vi "Import Configuration and Add Messages.vi"() -> ()   [LabVIEW 2020]
uses:
  <vilib>/addons/VeriStand Custom Device Scripting APIs/Instrument Addon/API/TypeDefs/Message Settings.ctl
  <vilib>/addons/VeriStand Custom Device Scripting APIs/Instrument Addon/API/TypeDefs/Protection Types.ctl
  <vilib>/addons/VeriStand Custom Device Scripting APIs/Instrument Addon/API/TypeDefs/Single Channel Format Settings.ctl
  <vilib>/addons/VeriStand Custom Device Scripting APIs/Instrument Addon/API/TypeDefs/Command Settings.ctl
  <vilib>/NI VeriStand/Custom Device API/Custom Device Item Ref.ctl
  <vilib>/addons/VeriStand Custom Device Scripting APIs/Instrument Addon/API/TypeDefs/Padding.ctl
  <vilib>/addons/VeriStand Custom Device Scripting APIs/Instrument Addon/API/TypeDefs/Array Type Cast Settings.ctl
  <vilib>/addons/VeriStand Custom Device Scripting APIs/Instrument Addon/API/TypeDefs/Array Element.ctl
  <vilib>/addons/VeriStand Custom Device Scripting APIs/Instrument Addon/Shared Directory/Type Cast Type.ctl
  <vilib>/addons/VeriStand Custom Device Scripting APIs/Instrument Addon/Shared Directory/Endian.ctl
  <vilib>/addons/VeriStand Custom Device Scripting APIs/Instrument Addon/API/Channels/Create Global MetaData Channel - Array - Type Cast.vi
  <vilib>/addons/VeriStand Custom Device Scripting APIs/Instrument Addon/API/Messages/Create Message - Value Change & Trigger.vi
  <vilib>/addons/VeriStand Custom Device Scripting APIs/Instrument Addon/API/Channels/Create MetaData Channel - Single Channel - Format.vi
  <vilib>/addons/VeriStand Custom Device Scripting APIs/Instrument Addon/API/Instrument Addon Scripting API.lvlib
  <vilib>/NI VeriStand/Custom Device API/Custom Device API.lvlib
  <vilib>/addons/VeriStand Custom Device Scripting APIs/Instrument Addon/Shared Directory/Instrument Addon Shared.lvlib
panel:
  in  "Configuration File to Import":path=path "Exported Configuration.dat"
  in  "Output System Definition File":path=path "System Definition Files/Import and Add Messages.nivssdf"
  in  "Input System Definition File":path=path "System Definition Files/Base.nivssdf"
  # "Overview: Demonstrate how to create an Instrument Addon Custom Device from a previously exported configuration and add additional messages and channels.\n\nNote: Must first run Basic Example.vi to generate the exported configuration .dat file used by this example.\n\nThe VI executes the following steps:\n1. Loads the exported configuration file from Basic Example.vi to create an Instrument Addon Custom Device with the same configuration.\n2. Adds a Global MetaData Channel and another message.\n3. For the new message, adds a Command Section and a MetaData Channel.\n4. Creates two linked channels by assigning the MetaData Channel refnum and the Global MetaData Channel refnum to two variable names in the command.\n5. Save System Definition file at the specification location.\n\nInstructions:\n1. Browse to the system definition file to be used as input.\n2. Browse to a path to save the system definition file as output. This may be the same as the input file.\n3. Browse to a path to import the previously exported custom device configuration from Basic Example.vi\n4. Run the VI and verify its results."
  # "System Definition Files"
  # "Configuration Files"
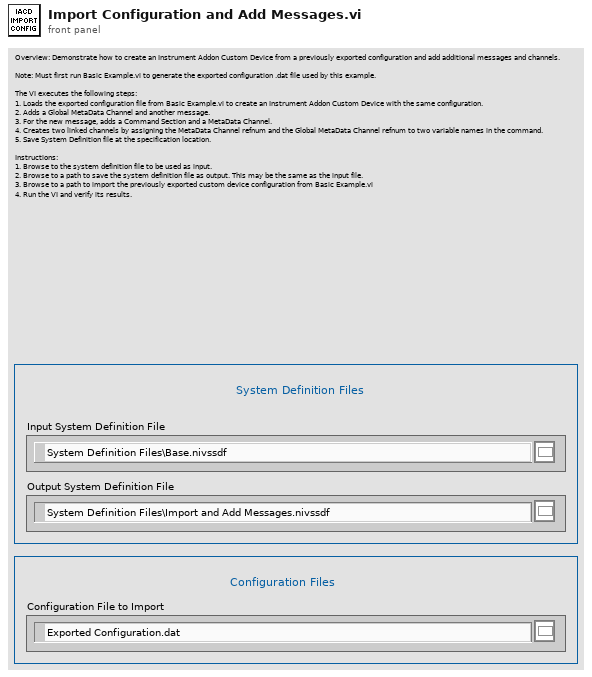
[diagram p1: front panel]
types:
  T1 = typedef "Custom Device API.lvlib/Custom Device Item Ref.ctl" = u64
  T2 = cluster{"Variable Name":string, "Channel Ref in":T1}
  T3 = typedef "Instrument Addon Scripting API.lvlib/Array Type Cast Settings.ctl" = cluster{"Elements":T4[], "Delimiter":string, "Type":T5, "Endian":T6}
  T4 = typedef "Instrument Addon Scripting API.lvlib/Array Element.ctl" = cluster{"Name":string, "Default Value":dbl, "Units":string}
  T5 = typedef "Instrument Addon Shared.lvlib/Type Cast Type.ctl" = enum16{"DBL", "SGL", "U64", "U32", "U16", "U8", "I64", "I32", "I16", "I8"}
  T6 = typedef "Instrument Addon Shared.lvlib/Endian.ctl" = enum16{"Native", "Little", "Big"}
  T7 = typedef "Instrument Addon Scripting API.lvlib/Padding.ctl" = cluster{"Pad Value":u8, "Length":u32}
  T8 = typedef "Instrument Addon Scripting API.lvlib/Command Settings.ctl" = cluster{"Command Format":string, "Linked Channels":cluster{"Variable Name":string, "Channel Ref in":T1}[], "Use Padding?":bool, "Padding":T7}
  T9 = typedef "Instrument Addon Scripting API.lvlib/Single Channel Format Settings.ctl" = cluster{"Format String":string, "Default Value":dbl, "Units":string}
  T10 = typedef "Instrument Addon Scripting API.lvlib/Message Settings.ctl" = cluster{"Protection":T11, "Enable Periodic Default":bool, "Trigger Channel refnum":u64}
  T11 = typedef "Instrument Addon Scripting API.lvlib/Protection Types.ctl" = enum16{"None", "CRC-32", "Checksum U16", "Checksum U32", "Checksum U8"}
  T12 = cluster{"Variable Name":string, "Channel Ref in":T1}[]
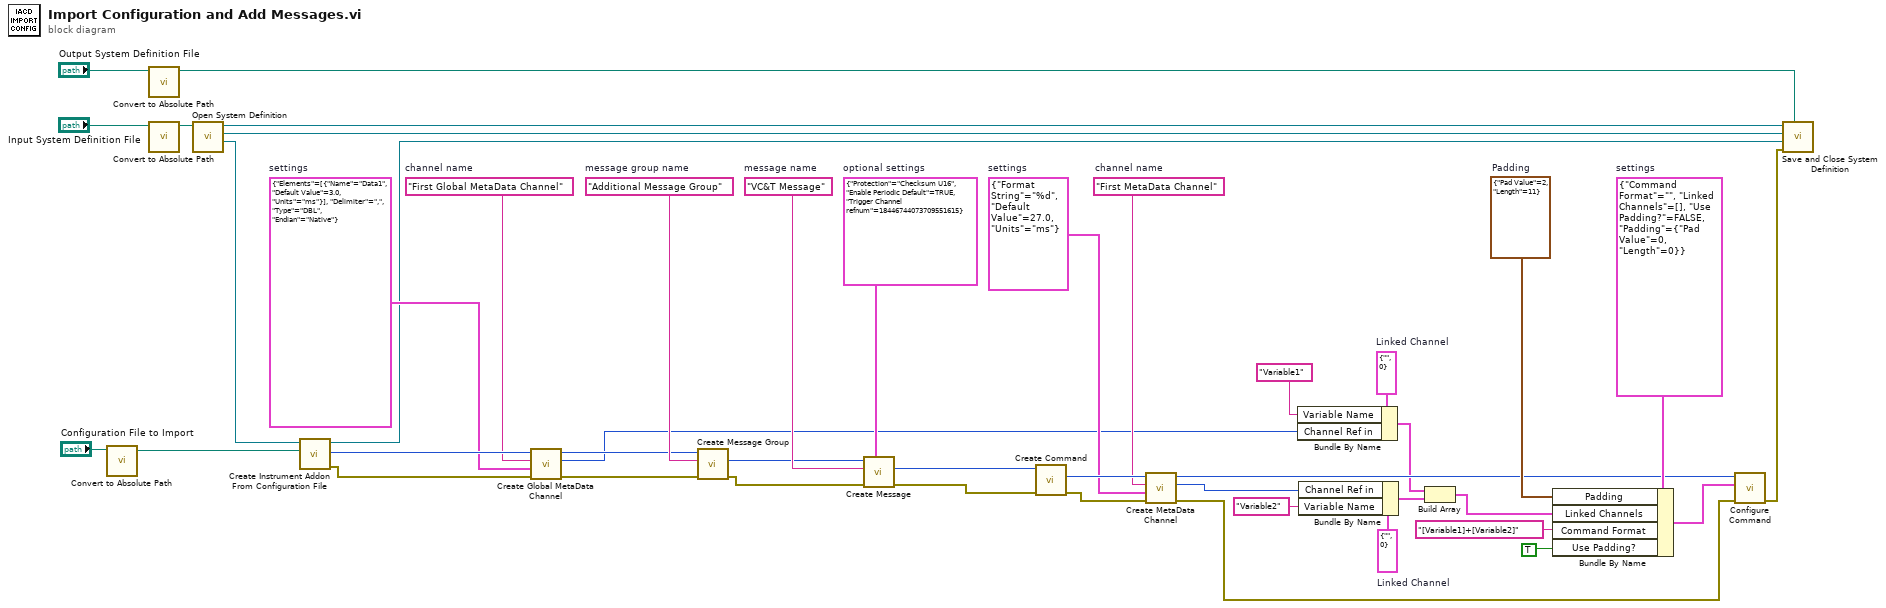
[diagram p0: block diagram]
diagram:
  w15 = T2 {"Variable Name"="", "Channel Ref in"=0}  # Linked Channel
  w16 = T3 {"Elements"=[{"Name"="Data1", "Default Value"=3.0, "Units"="ms"}], "Delimiter"=",", "Type"=enum."DBL", "Endian"=enum."Native"}  # settings
  w17 = "First Global MetaData Channel"  # channel name
  w27 = T7 {"Pad Value"=2, "Length"=11}  # Padding
  w33 = T2 {"Variable Name"="", "Channel Ref in"=0}  # Linked Channel
  w35 = T8 {"Command Format"="", "Linked Channels"=[], "Use Padding?"=FALSE, "Padding"={"Pad Value"=0, "Length"=0}}  # settings
  w37 = T9 {"Format String"="%d", "Default Value"=27.0, "Units"="ms"}  # settings
  w38 = "First MetaData Channel"  # channel name
  w41 = T10 {"Protection"=enum."Checksum U16", "Enable Periodic Default"=TRUE, "Trigger Channel refnum"=18446744073709551615}  # optional settings
  w43 = "VC&T Message"  # message name
  w44 = "Additional Message Group"  # message group name
  n1 = call "Convert to Absolute Path.vi"("System Definition File"="Configuration File to Import") -> ("Absolute Path"=w8:path)  [unwired: 10 in]
  n2 = call "Convert to Absolute Path.vi"("System Definition File"="Output System Definition File") -> ("Absolute Path"=w1:path)  [unwired: 10 in]
  n3 = call "Convert to Absolute Path.vi"("System Definition File"="Input System Definition File") -> ("Absolute Path"=w10:path)  [unwired: 10 in]
  n4 = call "Open System Definition.vi"("System Definition File"=w10) -> ("Target Refnum"=w7:refnum<k24>, "Root Refnum"=w3:refnum<k24>, "System Definition Refnum"=w2:refnum<k24>)  [unwired: 7 in, 1 out]
  n5 = call <vilib>:"Create Instrument Addon From Configuration File.vi"("configuration file path"=w8, "target in"=w7) -> ("error out"=w19:errorcluster, "instrument addon refnum"=w21:T1, "target out"=w4:refnum<k24>)  [unwired: 7 in]
  n6 = call-poly <vilib>:"Create Global MetaData Channel.vi"("error in (no error)"=w19, "settings"=w16, "channel name"=w17, "instrument addon refnum in"=w21) -> ("error out"=w18:errorcluster, "array refnum"=w12:T1, "instrument addon refnum out"=w20:T1)  [unwired: 4 in, 1 out]
  n7 = call <vilib>:"Create Message Group.vi"("error in (no error)"=w18, "message group name"=w44, "instrument addon refnum in"=w20) -> ("error out"=w40:errorcluster, "message group refnum out"=w42:T1)  [unwired: 6 in, 1 out]
  n8 = call-poly <vilib>:"Create Message.vi"("optional settings"=w41, "error in (no error)"=w40, "message name"=w43, "message group refnum in"=w42) -> ("error out"=w26:errorcluster, "message refnum out"=w25:T1)  [unwired: 5 in, 1 out]
  n9 = call <vilib>:"Create Command.vi"("error in"=w26, "message refnum In"=w25) -> ("error out"=w36:errorcluster, "command refnum"=w39:T1)  [unwired: 7 in, 1 out]
  n10 = call-poly <vilib>:"Create MetaData Channel.vi"("error in (no error)"=w36, "settings"=w37, "channel name"=w38, "command refnum in"=w39) -> ("error out"=w22:errorcluster, "channel refnum"=w29:T1, "command refnum out"=w24:T1)  [unwired: 5 in]
  n11 = Bundle By Name(cluster=w15, "Variable Name"="Variable1", "Channel Ref in"=w12) -> (w13:T2)
  n12 = Bundle By Name(cluster=w33, "Channel Ref in"=w29, "Variable Name"="Variable2") -> (w31:T2)
  n13 = Build Array(w13, w31) -> (w30:T12)
  n14 = Bundle By Name(cluster=w35, "Padding"=w27, "Linked Channels"=w30, "Command Format"="[Variable1]+[Variable2]", "Use Padding?"=TRUE) -> (w23:T8)
  n15 = call <vilib>:"Configure Command.vi"("error in (no error)"=w22, "settings"=w23, "command refnum in"=w24) -> ("error out"=w5:errorcluster)  [unwired: 7 in, 1 out]
  n16 = call "Save and Close System Definition.vi"("System Definition Path"=w1, "error in (no error)"=w5, "Target Refnum"=w4, "Root Refnum"=w3, "System Definition Refnum"=w2) -> ()  [unwired: 6 in, 1 out]
